vi "Sort Controls.vi"(11 "ConnRefs":refnum<vi>[](array[refnum])) -> (1 "TriggerRefs":refnum<vi>[](array[refnum]), 3 "AOAIRefs":T1[](array[typedef]))   [LabVIEW 2020, in "PXISlotGP.xctl"]
uses:
  PXISlotGP.xctl
  AOAIRefs.ctl
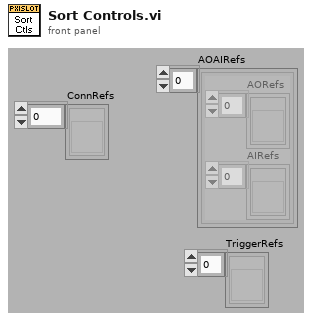
[diagram p1: front panel]
types:
  T1 = typedef "AOAIRefs.ctl" = cluster{"AORefs":refnum<vi>[], "AIRefs":refnum<vi>[]}
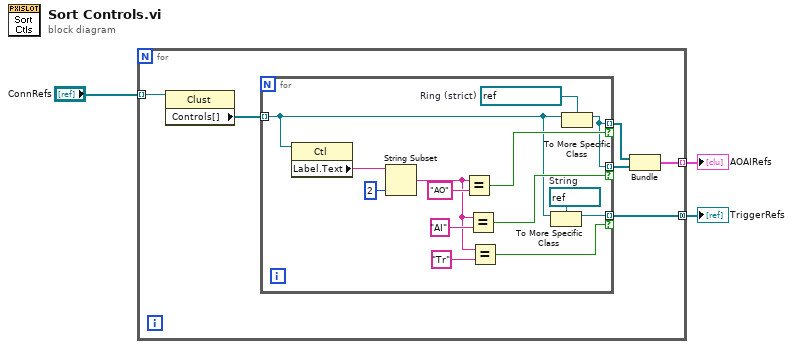
[diagram p0: block diagram]
diagram:
  n1 = for {
    tunnel: "ConnRefs" -> [w8] mode=indexing
    tunnel: [w7] -> w2 mode=concatenating
    tunnel: [w4] -> w1 mode=indexing
    n2 = property class="Clust"(reference=w8) -> ("Controls[]"=w9:refnum<vi>[])  [unwired: 1 in, 2 out]
    n3 = for {
      tunnel: w9 -> [w12] mode=indexing
      tunnel: [w11] -> w5 mode=indexing if=w20
      tunnel: [w11] -> w6 mode=indexing if=w18
      tunnel: [w14] -> w7 mode=indexing if=w15
      w10 = refnum<vi> refnum  # Ring (strict)
      w13 = refnum<vi> refnum  # String
      n4 = property class="Ctl"(reference=w12) -> ("Label.Text"=w22:string)  [unwired: 1 in, 2 out]
      n5 = String Subset(string=w22, length (rest)=2 ("length (rest)")) -> (substring=w16:string)  [unwired: 1 in]
      n6 = Equal?(x=w16, y="AO") -> (x = y?=w20:bool)
      n7 = Equal?(x=w16, y="AI") -> (x = y?=w18:bool)
      n8 = Equal?(x=w16, y="Tr") -> (x = y?=w15:bool)
      n9 = To More Specific Class(target class=w13, reference=w12) -> (specific class reference=w14:refnum<vi>)  [unwired: 1 in, 1 out]
      n10 = To More Specific Class(target class=w10, reference=w12) -> (specific class reference=w11:refnum<vi>)  [unwired: 1 in, 1 out]
    }
    n11 = Bundle(w5, w6) -> (w4:cluster{refnum<vi>[], refnum<vi>[]})  [unwired: 1 in]
  }
  "TriggerRefs" <- w2
  "AOAIRefs" <- w1
